vi "excel_rpt.vi"(0 "Pressure Data":string[][](array[string]), 3 "Supress Output":bool, 4 "Template Path":path, 5 "Average Flux Data":string[][](array[string])) -> ()   [LabVIEW 2015]
uses:
  <vilib>/addons/_office/excel.llb/Excel Easy Table (str).vi
  <vilib>/addons/_office/NI_ReportGenerationToolkit.lvlib
  <vilib>/Utility/NIReport.llb/Excel/NI_Excel.lvclass
  <vilib>/Utility/NIReport.llb/NI_report.lvclass
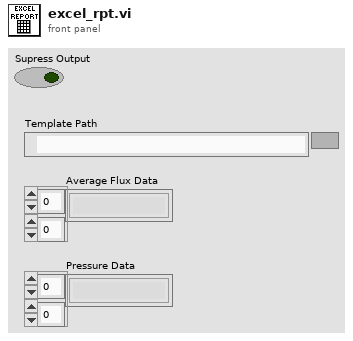
[diagram p1: front panel]
types:
  T1 = enum16{"Standard Report", "HTML", "Word", "Excel"}
  T2 = enum16{"maximized", "minimized", "normal", "no change"}
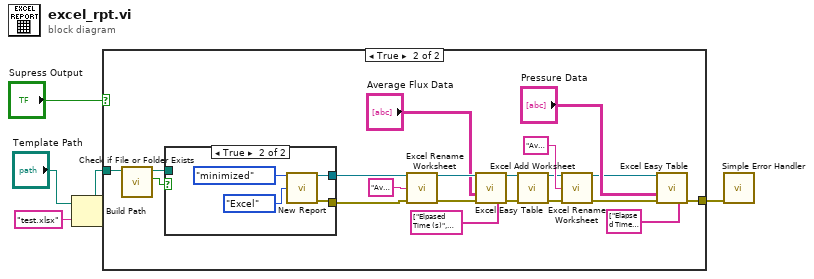
[diagram p0: block diagram]
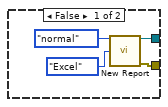
[diagram p3: hidden frame]
diagram:
  n1 = Build Path(base path="Template Path", name or relative path="test.xlsx") -> (appended path=w2:path)
  n2 = case shown="True" "Supress Output" {
    tunnel: w2 -> [_ w14]
    tunnel: [_ w7] -> w4
    frame False {
    }
    frame True {
      n3 = call <vilib>:"Check if File or Folder Exists.vi"("path"=w14) -> ("file or folder exists?"=w16:bool, "dup path"=w15:path)  [unwired: 8 in, 1 out]
      n4 = case shown="True" w16 {
        tunnel: [w29 w33] -> w8
        tunnel: w15 -> [_ _]
        tunnel: [w26 w30] -> w6
        frame False {
          n5 = call <vilib>:"New Report.vi"("window state (normal)"=T2."normal", "report type"=T1."Excel") -> ("report out"=w29:refnum<class "NI_report.lvclass">, "error out"=w26:errorcluster)  [unwired: 12 in]
        }
        frame True {
          n6 = call <vilib>:"New Report.vi"("window state (normal)"=T2."minimized", "report type"=T1."Excel") -> ("report out"=w33:refnum<class "NI_report.lvclass">, "error out"=w30:errorcluster)  [unwired: 12 in]
        }
      }
      n7 = call <vilib>:"Excel Rename Worksheet.vi"("report in"=w8, "worksheet name (\"\")"="Avg.  Flux" ("worksheet name (\"\")"), "error in (no error)"=w6) -> ("report out"=w11:refnum<class "NI_report.lvclass">, "error out"=w12:errorcluster)  [unwired: 11 in]
      n8 = call-poly <vilib>:"Excel Easy Table.vi"("report in"=w11, "text data"="Average Flux Data", "error in (no error)"=w12, "column headers"=string[] ["Elpased Time (s)", "Flow Rate (mL/min)", "Flux (L/h/m²)"]) -> ("report out"=w17:refnum<class "NI_report.lvclass">, "error out"=w18:errorcluster)  [unwired: 7 in, 3 out]
      n9 = call <vilib>:"Excel Add Worksheet.vi"("report in"=w17, "error in (no error)"=w18) -> ("report out"=w19:refnum<class "NI_report.lvclass">, "error out"=w20:errorcluster)  [unwired: 12 in]
      n10 = call <vilib>:"Excel Rename Worksheet.vi"("report in"=w19, "worksheet name (\"\")"="Avg. Pressure" ("worksheet name (\"\")"), "error in (no error)"=w20) -> ("report out"=w21:refnum<class "NI_report.lvclass">, "error out"=w22:errorcluster)  [unwired: 11 in]
      n11 = call-poly <vilib>:"Excel Easy Table.vi"("report in"=w21, "text data"="Pressure Data", "error in (no error)"=w22, "column headers"=string[] ["Elapsed Time (s)", "Pressure (PSIG)"]) -> ("error out"=w7:errorcluster)  [unwired: 7 in, 4 out]
    }
  }
  n12 = call <vilib>:"Simple Error Handler.vi"("error in (no error)"=w4) -> ()  [unwired: 4 in, 5 out]
